vi "Save.vi"(9 "Notatka":string, 10 "Tytuł":string, 11 "ProgramData in":T1={"Tytuły"=[], "Folder"=path "", "Data/tytul"=[], "Ostatni index"=-10, "Title"="", "Note"=""}) -> (3 "ProgramData out":T1={"Tytuły"=[], "Folder"=path "", "Data/tytul"=[], "Ostatni index"=-10, "Title"="", "Note"=""})   [LabVIEW 2020]
uses:
  #typeDef_ProgramData.ctl
panel:
  in  "Notatka 2":string
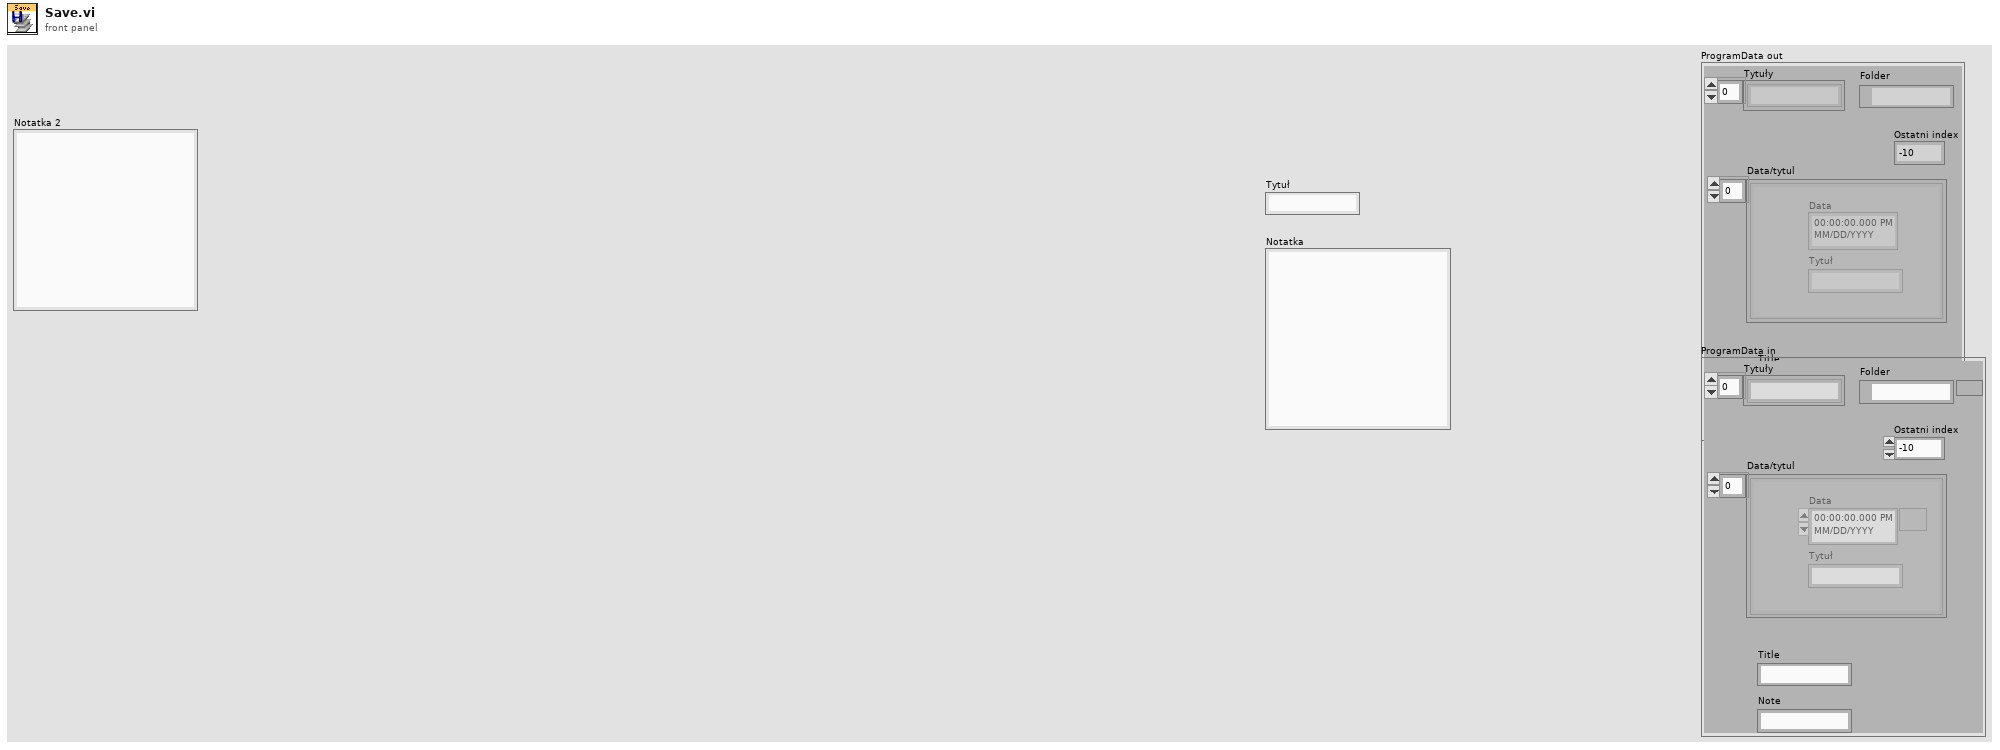
[diagram p1: front panel]
types:
  T1 = typedef "#typeDef_ProgramData.ctl" = cluster{"Tytuły":string[], "Folder":path, "Data/tytul":cluster{"Data":timestamp, "Tytuł":string}[], "Ostatni index":i32, "Title":string, "Note":string}
  T2 = enum16{"open", "replace", "create", "open or create", "replace or create", "replace or create with confirmation"}
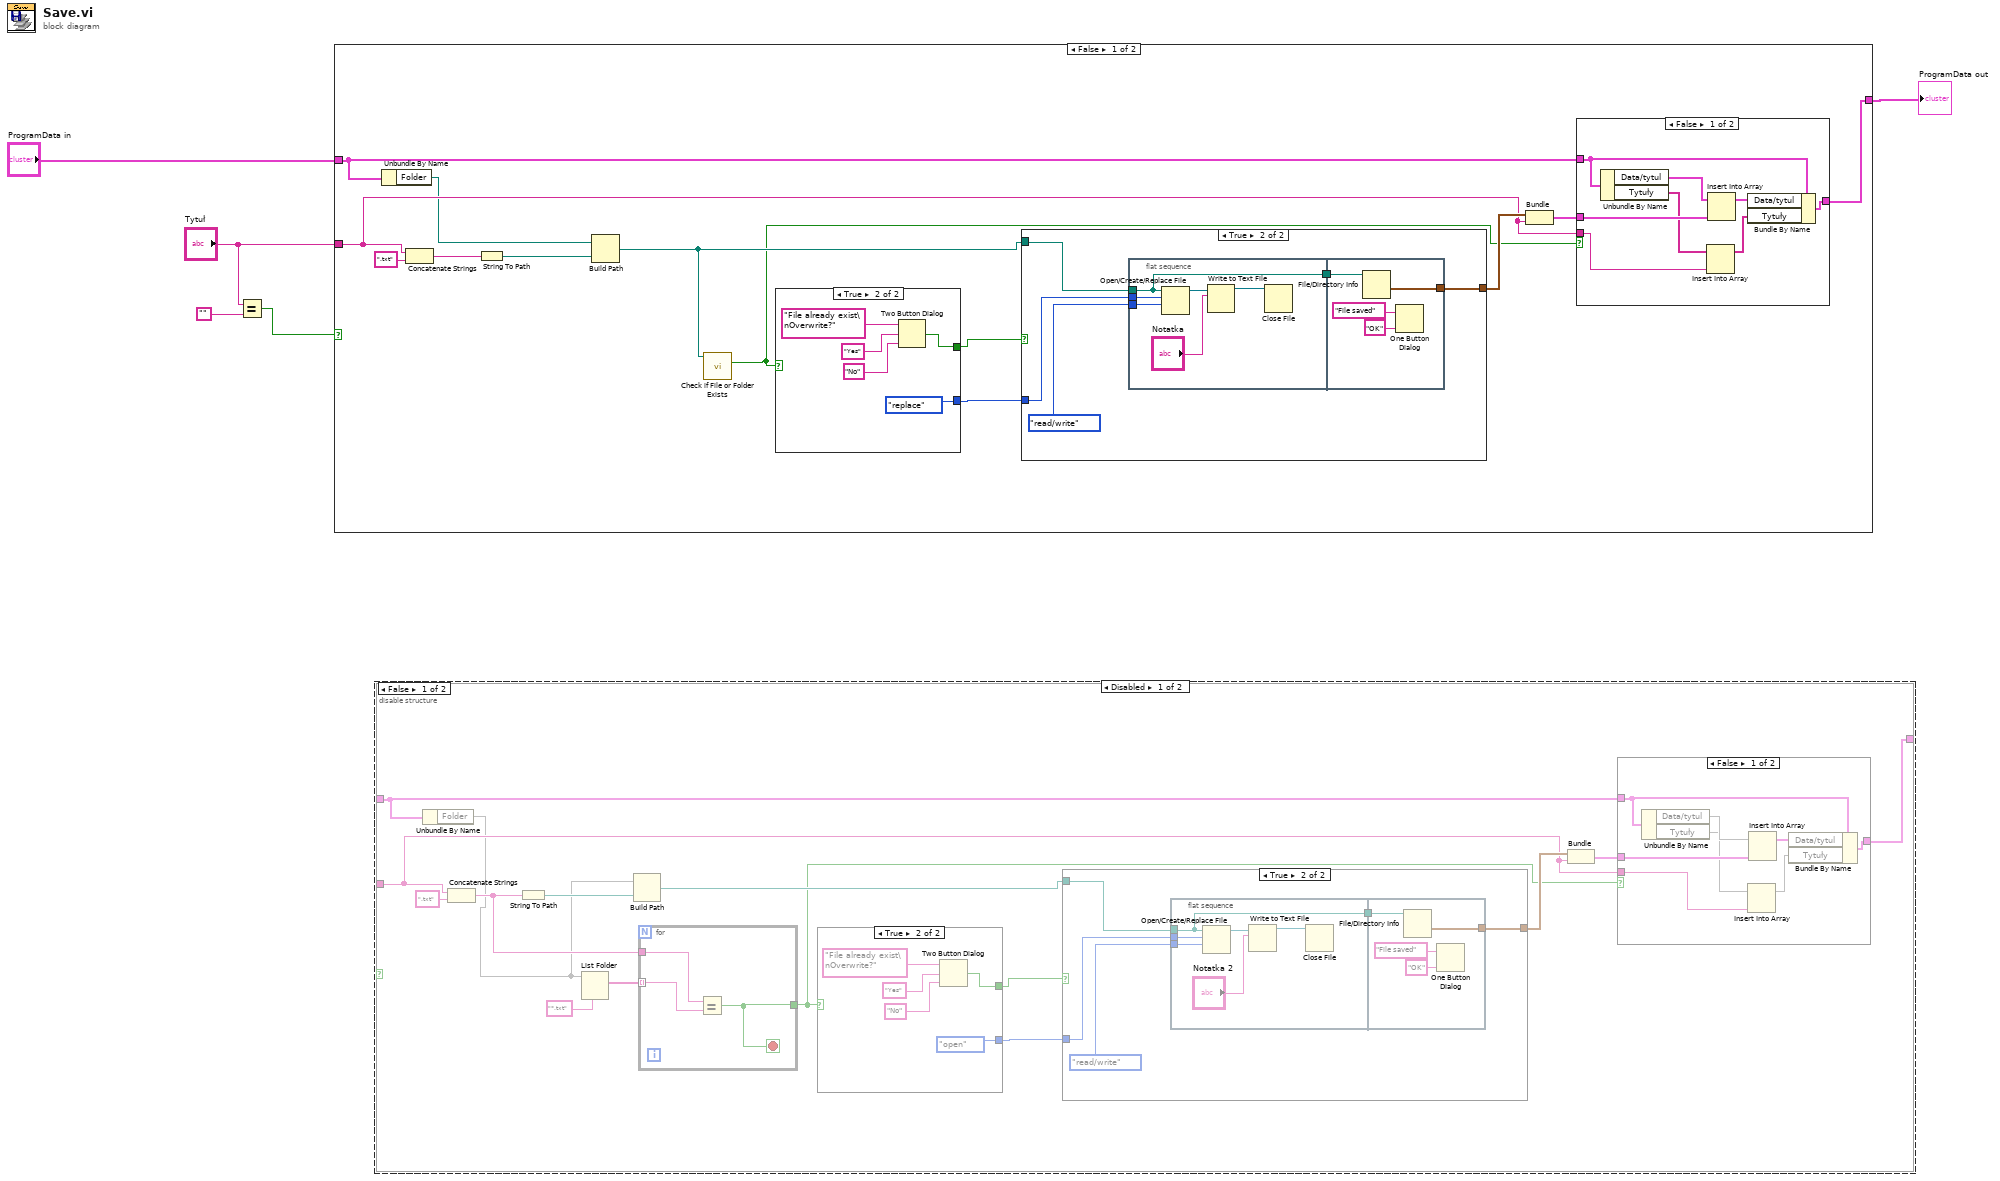
[diagram p0: block diagram]
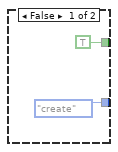
[diagram p2: hidden frame]
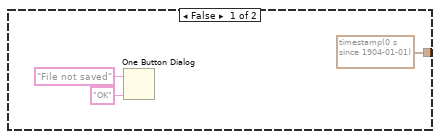
[diagram p4: hidden frame]
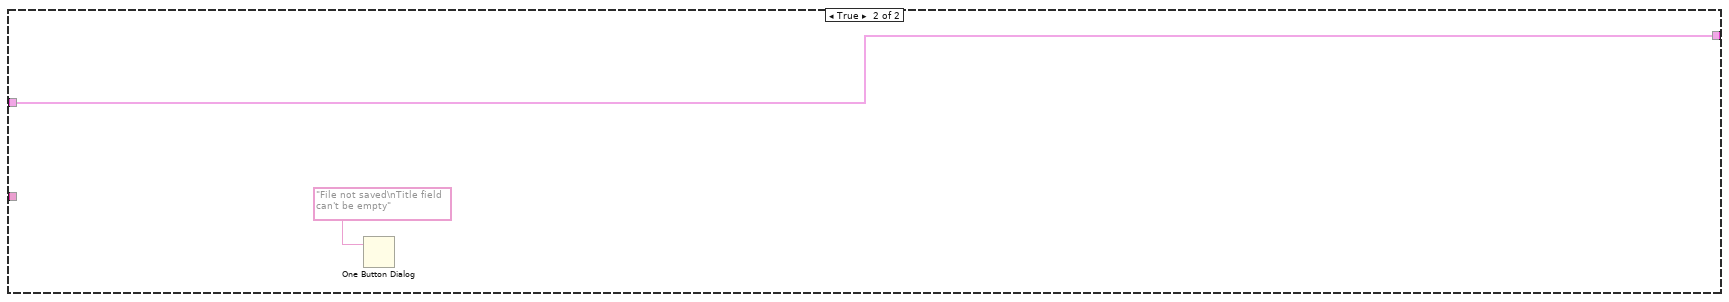
[diagram p5: hidden frame]
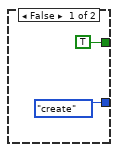
[diagram p7: hidden frame]
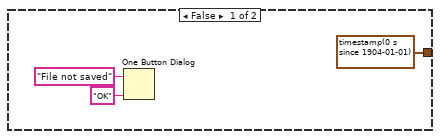
[diagram p9: hidden frame]
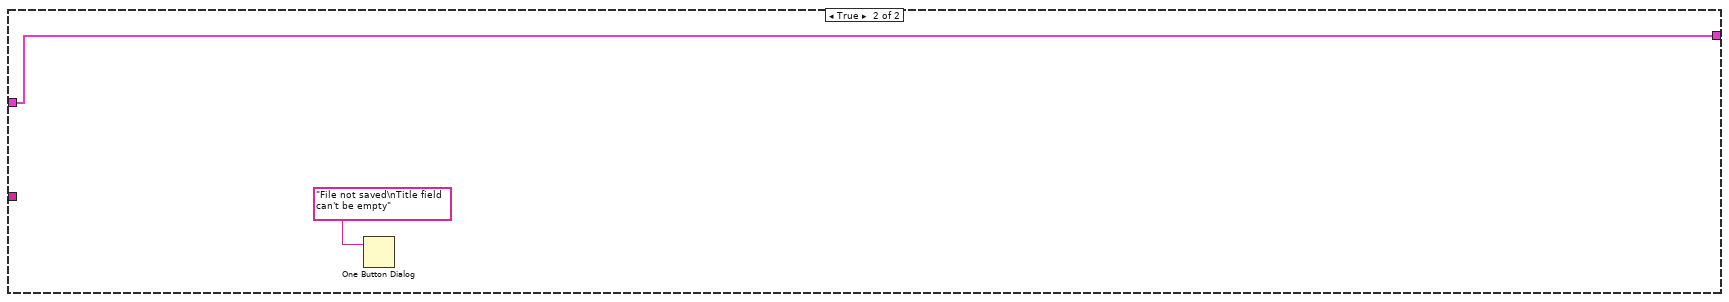
[diagram p10: hidden frame]
diagram:
  n1 = Equal?(x="Tytuł", y="") -> (x = y?=w1:bool)
  n2 = case shown="False" w1 {
    tunnel: "Tytuł" -> [w11 _]
    tunnel: "ProgramData in" -> [w16 w53]
    tunnel: [w15 w53] -> w4
    frame False {
      n3 = Unbundle By Name(w16) -> ("Folder"=w10:path)
      n4 = Concatenate Strings(w11, ".txt" ("string")) -> (w14:string)
      n5 = String To Path(string=w14) -> (path=w13:path)
      n6 = Build Path(base path=w10, name or relative path=w13) -> (appended path=w7:path)
      n7 = call <vilib>:"Check if File or Folder Exists.vi"("path"=w7) -> ("file or folder exists?"=w6:bool)  [unwired: 8 in, 2 out]
      n8 = case shown="True" w6 {
        tunnel: [TRUE ("T button?") w22] -> w8
        tunnel: [T2."create" ("operation (0:open)") T2."replace" ("operation (0:open)")] -> w9
        frame False {
        }
        frame True {
          n9 = Two Button Dialog(message="File already exist\nOverwrite?", 1:"No" ("F button name (\"Cancel\")"), 2:"Yes" ("T button name (\"OK\")")) -> (T button?=w22:bool)
        }
      }
      n10 = case shown="True" w8 {
        tunnel: w9 -> [_ w41]
        tunnel: w7 -> [_ w40]
        tunnel: [timestamp(0 s since 1904-01-01) ("last mod") w38] -> w18
        frame False {
          n11 = One Button Dialog(message="File not saved", button name ("OK")="OK") -> ()  [unwired: 1 out]
        }
        frame True {
          n12 = flat-sequence {
            tunnel: enum16{"read/write", "read-only", "write-only"}."read/write" ("access (0:read/write)") -> [w48]
            tunnel: w41 -> [w46]
            tunnel: w40 -> [w44]
            tunnel: [w44] -> w39
            tunnel: w39 -> [w52]
            tunnel: [w49] -> w38
            frame #0 {
              n13 = Open/Create/Replace File(file path (use dialog)=w44, operation (0:open)=w46, access (0:read/write)=w48) -> (refnum out=w47:refnum<file>)  [unwired: 3 in, 2 out]
              n14 = Write to Text File(file (use dialog)=w47, text="Notatka") -> (refnum out=w45:refnum<file>)  [unwired: 2 in, 2 out]
              n15 = Close File(refnum=w45) -> ()  [unwired: 1 in, 2 out]
            }
            frame #1 {
              n16 = File/Directory Info(path=w52) -> (last mod=w49:timestamp)  [unwired: 1 in, 6 out]
              n17 = One Button Dialog(message="File saved", button name ("OK")="OK") -> ()  [unwired: 1 out]
            }
          }
        }
      }
      n18 = Bundle("last mod"=w18, "Tytuł"=w11) -> (w17:cluster{"last mod":timestamp, "Tytuł":string})  [unwired: 1 in]
      n19 = case shown="False" w6 {
        tunnel: w17 -> [w33 _]
        tunnel: w16 -> [w31 w34]
        tunnel: [w29 w34] -> w15
        tunnel: w11 -> [w26 _]
        frame False {
          n20 = Unbundle By Name(w31) -> ("Data/tytul"=w32:cluster{"Data":timestamp, "Tytuł":string}[], "Tytuły"=w27:string[])
          n21 = Insert Into Array(array=w27, new element=w26) -> (w28:string[])  [unwired: 1 in]
          n22 = Insert Into Array(array=w32, new element=w33) -> (w30:cluster{"Data":timestamp, "Tytuł":string}[])  [unwired: 1 in]
          n23 = Bundle By Name(cluster=w31, "Data/tytul"=w30, "Tytuły"=w28) -> (w29:T1)
        }
        frame True {
        }
      }
    }
    frame True {
      n24 = One Button Dialog(message="File not saved\nTitle field can't be empty") -> ()  [unwired: 1 in, 1 out]
    }
  }
  "ProgramData out" <- w4
  n25 = disable-structure shown="Disabled" {
    frame Disabled {
      n26 = case shown="False" {
        selector: _ -> [_ _]
        tunnel: _ -> [w60 _]
        tunnel: _ -> [w67 w107]
        tunnel: [w66 w107] -> _
        frame False {
          n27 = Unbundle By Name(w67) -> ("Folder"=w59)
          n28 = Concatenate Strings(w60, ".txt" ("string")) -> (w64:string)
          n29 = String To Path(string=w64) -> (path=w63:path)
          n30 = List Folder(path=w59, pattern="*.txt") -> (filenames=w65:string[])  [unwired: 2 in, 3 out]
          n31 = Build Path(base path=w59, name or relative path=w63) -> (appended path=w57:path)
          n32 = for {
            tunnel: w65 -> [w78] mode=indexing
            tunnel: w64 -> [w79]
            tunnel: [w77] -> w55
            stop <- w77 stop-if-true
            n33 = Equal?(x=w79, y=w78) -> (x = y?=w77:bool)
          }
          n34 = case shown="True" w55 {
            tunnel: [TRUE ("T button?") w73] -> w56
            tunnel: [T2."create" ("operation (0:open)") T2."open" ("operation (0:open)")] -> w58
            frame False {
            }
            frame True {
              n35 = Two Button Dialog(message="File already exist\nOverwrite?", 1:"No" ("F button name (\"Cancel\")"), 2:"Yes" ("T button name (\"OK\")")) -> (T button?=w73:bool)
            }
          }
          n36 = case shown="True" w56 {
            tunnel: w58 -> [_ w95]
            tunnel: w57 -> [_ w94]
            tunnel: [timestamp(0 s since 1904-01-01) ("last mod") w92] -> w69
            frame False {
              n37 = One Button Dialog(message="File not saved", button name ("OK")="OK") -> ()  [unwired: 1 out]
            }
            frame True {
              n38 = flat-sequence {
                tunnel: enum16{"read/write", "read-only", "write-only"}."read/write" ("access (0:read/write)") -> [w102]
                tunnel: w95 -> [w100]
                tunnel: w94 -> [w98]
                tunnel: [w98] -> w93
                tunnel: w93 -> [w106]
                tunnel: [w103] -> w92
                frame #0 {
                  n39 = Open/Create/Replace File(file path (use dialog)=w98, operation (0:open)=w100, access (0:read/write)=w102) -> (refnum out=w101:refnum<file>)  [unwired: 3 in, 2 out]
                  n40 = Write to Text File(file (use dialog)=w101, text="Notatka 2") -> (refnum out=w99:refnum<file>)  [unwired: 2 in, 2 out]
                  n41 = Close File(refnum=w99) -> ()  [unwired: 1 in, 2 out]
                }
                frame #1 {
                  n42 = File/Directory Info(path=w106) -> (last mod=w103:timestamp)  [unwired: 1 in, 6 out]
                  n43 = One Button Dialog(message="File saved", button name ("OK")="OK") -> ()  [unwired: 1 out]
                }
              }
            }
          }
          n44 = Bundle("last mod"=w69, w60) -> (w68:cluster{"last mod":timestamp, void})  [unwired: 1 in]
          n45 = case shown="False" w55 {
            tunnel: w68 -> [w87 _]
            tunnel: w67 -> [w85 w88]
            tunnel: [w83 w88] -> w66
            tunnel: w60 -> [w80 _]
            frame False {
              n46 = Unbundle By Name(w85) -> ("Data/tytul"=w86, "Tytuły"=w81)
              n47 = Insert Into Array(array=w81, new element=w80) -> (w82)  [unwired: 1 in]
              n48 = Insert Into Array(array=w86, new element=w87) -> (w84:cluster{"last mod":timestamp, void}[])  [unwired: 1 in]
              n49 = Bundle By Name(cluster=w85, "Data/tytul"=w84, "Tytuły"=w82) -> (w83:cluster{})
            }
            frame True {
            }
          }
        }
        frame True {
          n50 = One Button Dialog(message="File not saved\nTitle field can't be empty") -> ()  [unwired: 1 in, 1 out]
        }
      }
    }
    frame Enabled {
    }
  }
